vi "Read Transconductance.vi"   [LabVIEW 2020, in "Keithley 2600 Series.lvlib"]
doc: "Performs a source sweep and calculates the transconductance."
uses:
  <instrlib>/Keithley 2600 Series/Keithley 2600 Series.lvlib
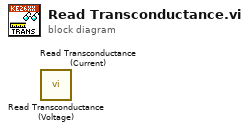
[diagram p0: block diagram]
diagram:
  n1 = call <instrlib>:"Read Transconductance (Voltage).vi"() -> ()  [unwired: 11 in, 5 out]
  n2 = call <instrlib>:"Read Transconductance (Current).vi"() -> ()  [unwired: 11 in, 5 out]
